vi "Read Active Dot.vi"(8 "error in (no error)":errorcluster, 11 "Setting Database in":refnum<class "Setting Database.lvclass">) -> (0 "error out":errorcluster, 2 "Active Dot":refnum<class "Dot Settings.lvclass">, 3 "Setting Database out":refnum<class "Setting Database.lvclass">)   [LabVIEW 2019, in "Setting Database.lvclass"]
uses:
  Setting Database.lvclass
  Dot Settings/Dot Settings.lvclass
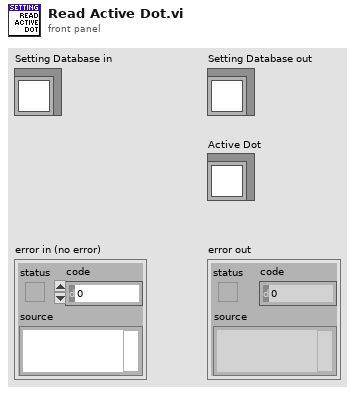
[diagram p1: front panel]
types:
  T1 = cluster{"Path":i32, "Funnel":i32, "Rectangle":i32, "Dot":i32}
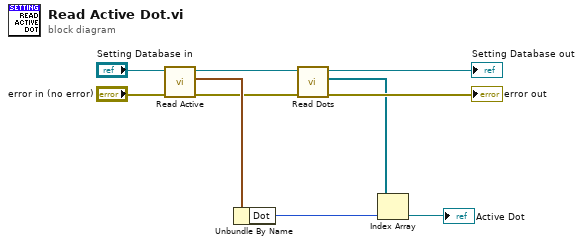
[diagram p0: block diagram]
diagram:
  n1 = call "Read Active.vi"("error in (no error)"="error in (no error)", "Setting Database in"="Setting Database in") -> ("error out"=w5:errorcluster, "Active"=w7:T1, "Setting Database out"=w8:refnum<class "Setting Database.lvclass">)  [unwired: 7 in]
  n2 = Unbundle By Name(w7) -> ("Dot"=w6:i32)
  n3 = call "Read Dots.vi"("error in (no error)"=w5, "Setting Database in"=w8) -> ("error out"=→"error out":errorcluster, "Dots"=w1:refnum<class "Dot Settings.lvclass">[], "Setting Database out"=→"Setting Database out":refnum<class "Setting Database.lvclass">)  [unwired: 7 in]
  n4 = Index Array(array=w1, index=w6) -> (element=→"Active Dot":refnum<class "Dot Settings.lvclass">)
